vi "Save VI For Previous Version.vi"(8 "Error In":errorcluster, 9 "LabVIEW Version":T1, 10 "Save Path":path, 11 "VI Path":path) -> (0 "Error Out":errorcluster, 2 "Warnings":string)   [LabVIEW 2020, in "LMH-Toolbox.lvlib" / "LMH-VITools.lvlib"]
uses:
  LMH-VITools.lvlib
  Type Defs/LabVIEW Version.ctl
  LMH-Toolbox.lvlib
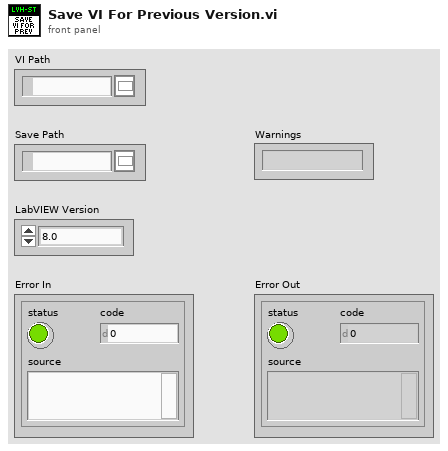
[diagram p1: front panel]
types:
  T1 = typedef "LMH-Toolbox.lvlib/LabVIEW Version.ctl" = enum16{"8.0", "8.2", "8.6", "9.0", "10.0", "11.0", "12.0", "13.0"}
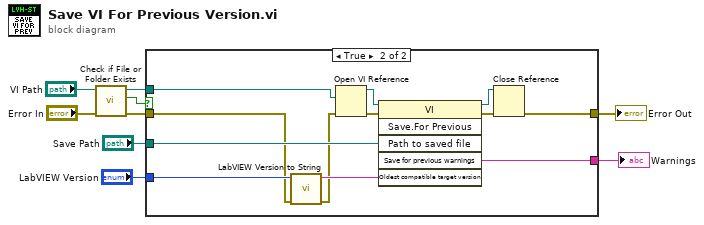
[diagram p0: block diagram]
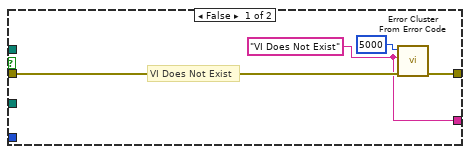
[diagram p2: hidden frame]
diagram:
  n1 = call <vilib>:"Check if File or Folder Exists.vi"("error in (no error)"="Error In", "path"="VI Path") -> ("error out"=w5:errorcluster, "file or folder exists?"=w7:bool, "dup path"=w6:path)  [unwired: 7 in]
  n2 = case shown="True" w7 {
    tunnel: w6 -> [_ w23]
    tunnel: w5 -> [w12 w14]
    tunnel: "Save Path" -> [_ w22]
    tunnel: [w13 w19] -> w3
    tunnel: [w10 w18] -> w2
    tunnel: "LabVIEW Version" -> [_ w16]
    frame False {
      w10 = "VI Does Not Exist" ("error message (\"\")")
      # "VI Does Not Exist"
      n3 = call <vilib>:"Error Cluster From Error Code.vi"("error in (no error)"=w12, "error message (\"\")"=w10, "error code (0)"=5000) -> ("error out"=w13:errorcluster)  [unwired: 6 in]
    }
    frame True {
      n4 = call "LabVIEW Version to String.vi"("Error In"=w14, "LabVIEW Version"=w16) -> ("Error Out"=w15:errorcluster, "LabVIEW Version"=w17:string)  [unwired: 8 in]
      n5 = Open VI Reference(vi path=w23, error in (no error)=w15) -> (vi reference=w25:refnum<vi>, error out=w24:errorcluster)  [unwired: 4 in]
      n6 = invoke class="VI" method="Save.For Previous"(reference=w25, error in=w24, "Path to saved file"=w22, "Oldest compatible target version"=w17) -> (reference out=w20:refnum<vi>, error out=w21:errorcluster, "Save for previous warnings"=w18:string)  [unwired: 2 in, 3 out]
      n7 = Close Reference(reference=w20, error in (no error)=w21) -> (error out=w19:errorcluster)
    }
  }
  "Error Out" <- w3
  "Warnings" <- w2
